vi "Titelsteuerung.vi"(2 "time-string":string, 3 "titel":string, 4 "Pause":bool) -> (0 "String":string)   [LabVIEW 2012]
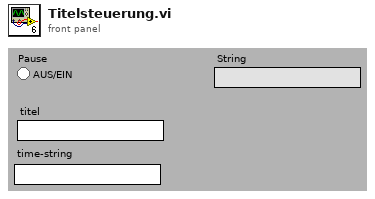
[diagram p1: front panel]
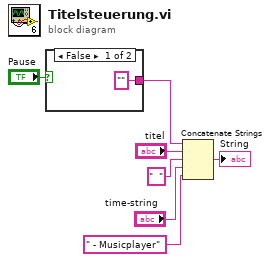
[diagram p0: block diagram]
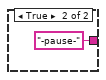
[diagram p2: hidden frame]
diagram:
  n1 = case shown="False" "Pause" {
    tunnel: ["" "-pause-"] -> w6
    frame False {
    }
    frame True {
    }
  }
  n2 = Concatenate Strings(w6, "titel", "  " ("String"), "time-string", " - Musicplayer" ("String")) -> (→"String":string)
